vi "recover_phase.vi"(9 "Normalized transmission (r=wl, c=v)":dbl[][](array[numeric]), 10 "Extrema (type, idx)":T1(array[cluster])) -> (1 "Phase (r=wl, c=v)":dbl[][](array[numeric]))   [LabVIEW 2019]
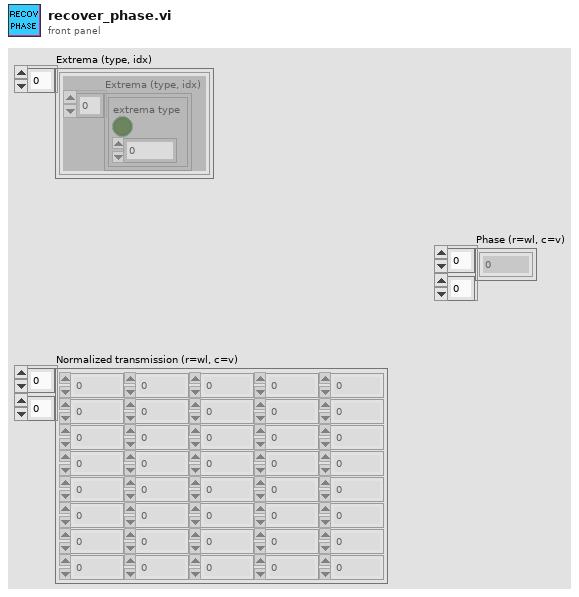
[diagram p1: front panel]
types:
  T1 = cluster{"Extrema (type, idx)":cluster{"extrema type":bool, i32}[]}[]
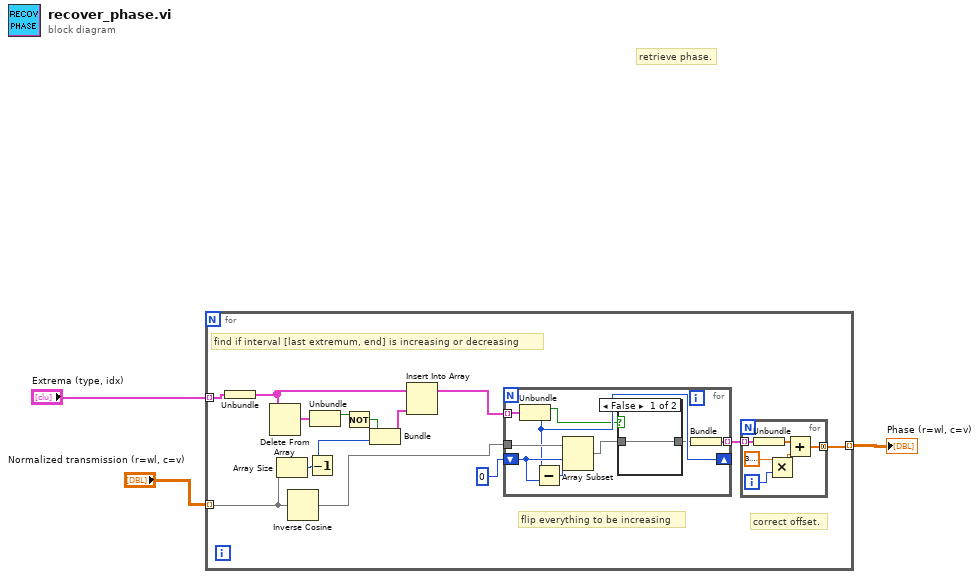
[diagram p0: block diagram]
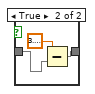
[diagram p2: hidden frame]
diagram:
  # "retrieve phase."
  n1 = for {
    tunnel: [w4] -> w3 mode=indexing
    tunnel: "Normalized transmission (r=wl, c=v)" -> [w17] mode=indexing
    tunnel: "Extrema (type, idx)" -> [w9] mode=indexing
    # "correct offset."
    # "flip everything to be increasing"
    # "find if interval [last extremum, end] is increasing or decreasing"
    n2 = Unbundle(w9) -> ("Extrema (type, idx)"=w8:cluster{"extrema type":bool, i32}[])
    n3 = Delete From Array(array=w8) -> (deleted portion=w14:cluster{"extrema type":bool, i32})  [unwired: 2 in, 1 out]
    n4 = Array Size(array=w17) -> (size(s)=w16:i32)
    n5 = Inverse Cosine(1:w17) -> (0:w13:dbl[])
    n6 = Decrement(x=w16) -> (x-1=w15:i32)
    n7 = Unbundle(w14) -> ("extrema type"=w12:bool)  [unwired: 1 out]
    n8 = Not(x=w12) -> (.not. x?=w11:bool)
    n9 = Bundle(w11, w15) -> (w10:cluster{bool, i32})  [unwired: 1 in]
    n10 = Insert Into Array(array=w8, new element=w10) -> (w7:cluster{"extrema type":bool, i32}[])  [unwired: 1 in]
    n11 = for {
      tunnel: w7 -> [w31] mode=indexing
      tunnel: w13 -> [w32]
      shift-right: [w28] -> _
      shift-left: 0 -> [w30]
      tunnel: [w24] -> w5 mode=indexing
      n12 = Unbundle(w31) -> ("extrema type"=w27:bool, w28:i32)
      n13 = Subtract(x=w28, y=w30) -> (x-y=w29:i32)
      n14 = Array Subset(array=w32, index=w30, length=w29) -> (w26:dbl[])
      n15 = case shown="False" w27 {
        tunnel: w26 -> [w33 w35]
        tunnel: [w33 w36] -> w25
        frame False {
        }
        frame True {
          n16 = Subtract(x=3.141592653589793, y=w35) -> (x-y=w36:dbl[])
        }
      }
      n17 = Bundle(w25) -> (w24:cluster{dbl[]})  [unwired: 1 in]
    }
    n18 = for {
      tunnel: w5 -> [w19] mode=indexing
      tunnel: [w22] -> w4 mode=concatenating
      i -> [w23]
      n19 = Unbundle(w19) -> (w18:dbl[])
      n20 = Multiply(x=3.141592653589793, y=w23) -> (x*y=w21:dbl)
      n21 = Add(x=w18, y=w21) -> (x+y=w22:dbl[])
    }
  }
  "Phase (r=wl, c=v)" <- w3
